vi "Homing.vi"(7 "Offset Home 2 RCM":dbl[](array[numeric])=[0.0, 0.0, 0.0, 0.0], 8 "error in":errorcluster, 9 "Stage PID Cluster":T2={"Stage Z PID"={"Kp"=0.0005, "Kd"=0.001, "Ki"=0.0}, "Stage Y PID"={"Kp"=0.0003, "Kd"=0.01, "Ki"=0.0}, "Stage X PID"={"Kp"=0.0003, "Kd"=0.01, "Ki"=0.0}}, 10 "L1 to L4 PID Cluster":T1={"L1 PID Gains"={"Kp"=0.005, "Kd"=0.5, "Ki"=0.0005}, "L2 PID Gains"={"Kp"=0.01, "Kd"=1.0, "Ki"=0.005}, "L3 PID Gains"={"Kp"=0.05, "Kd"=1.0, "Ki"=0.0005}, "L4 PID Gains"={"Kp"=0.1, "Kd"=0.1, "Ki"=0.0005}}, 11 "FPGA VI Reference In":refnum<k20>) -> (0 "error out":errorcluster, 1 "Last Stage Posit":dbl[](array[numeric]), 2 "Last L1 to L4 Posit":dbl[](array[numeric]), 3 "FPGA VI Reference Out":refnum<k20>)   [LabVIEW 2016]
uses:
  <vilib>/Platform/TimedLoop/XDataNode/timing_clust.ctl
  <vilib>/Platform/TimedLoop/XDataNode/nitl_modes.ctl
  <vilib>/Platform/TimedLoop/XDataNode/wakeup.ctl
  Library/KevinLibraryAll/labview2010/kevLib2010/Simple Filters/kDelay.vi
  Global Variables.vi
  <vilib>/Utility/error.llb/Error Cluster From Error Code.vi
  <vilib>/rvi/errors/niLvFpgaAdjustHostInterfaceError.vi
  <vilib>/platform/TimedLoop/XDataNode/XDataNode.xnode
  <vilib>/rvi/interface/nirviReadWriteControl/nirviReadWriteControl.xnode
  FPGA Bitfiles/PhantomControlPI_FPGATarget_QuadCtr2_E2412E44.lvbitx
  IRISS_FPGA_IO.vi
  <vilib>/Platform/TimedLoop/XDataNode/XDNodeRunTimeDep.lvlib
  Library/KevinLibraryAll/labview2010/kevLib2010.lvlib
  Library/KevinLibraryAll/labview2011/kevLib2011.lvlib
  Library/KevinLibraryAll/labview/KevLib01.lvlib
  Library/jmslib.lvlib
  NiFpgaLv.dll
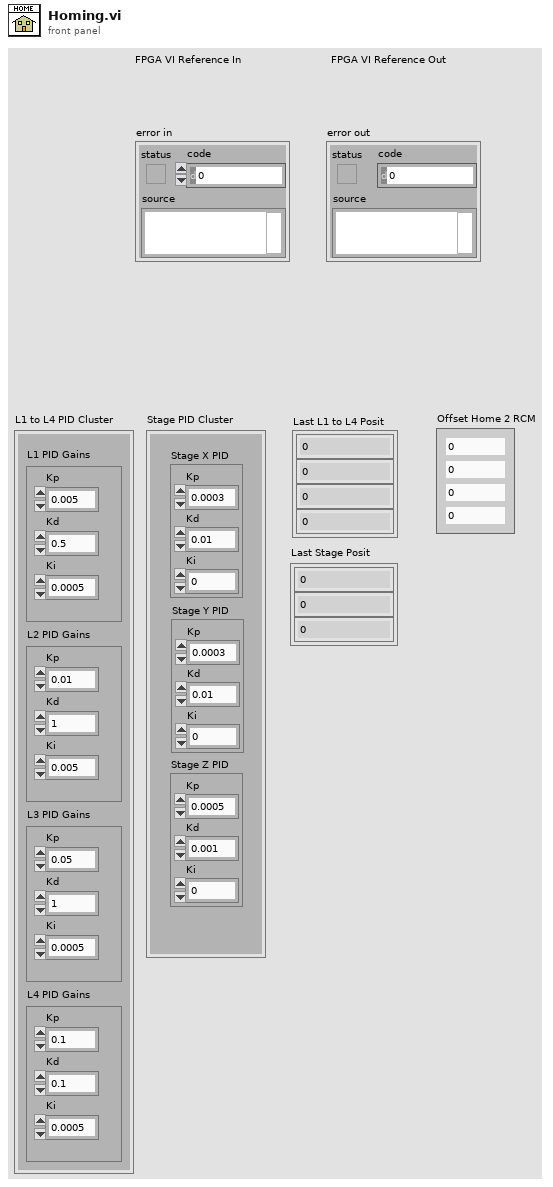
[diagram p1: front panel]
types:
  T1 = cluster{"L1 PID Gains":cluster{"Kp":dbl, "Kd":dbl, "Ki":dbl}, "L2 PID Gains":cluster{"Kp":dbl, "Kd":dbl, "Ki":dbl}, "L3 PID Gains":cluster{"Kp":dbl, "Kd":dbl, "Ki":dbl}, "L4 PID Gains":cluster{"Kp":dbl, "Kd":dbl, "Ki":dbl}}
  T2 = cluster{"Stage Z PID":cluster{"Kp":dbl, "Kd":dbl, "Ki":dbl}, "Stage Y PID":cluster{"Kp":dbl, "Kd":dbl, "Ki":dbl}, "Stage X PID":cluster{"Kp":dbl, "Kd":dbl, "Ki":dbl}}
  T3 = typedef "XDNodeRunTimeDep.lvlib/timing_clust.ctl" = cluster{"Expected End [f-1]":u64, "Actual End [f-1]":u64, "Finished Late? [f-1]":bool, "Expected End [i-1]":u64, "Actual End [i-1]":u64, "Finished Late? [i-1]":bool, "Expected Start [i]":u64, "Actual Start [i]":u64, "Expected Start [f]":u64, "Actual Start [f]":u64, "Source Name":string, "Structure Name":string, "Period":i64, "Deadline":i64, "Offset":i64, "Start":i64, "Priority":i32, "Timeout":i32, "Mode":T4, "Wakeup Reason":T5, "Error":errorcluster, "Source Type":string, "Secondary Source Type":string, "Global End Time":u64, "Global Start Time":u64, "Frame Duration":u64, "Iteration Duration":u64, "Assigned CPU":i32, "I/O Scan Engine Mode":u32}
  T4 = typedef "XDNodeRunTimeDep.lvlib/nitl_modes.ctl" = enum32{"No Change", "Process missed periods, maintain original phase", "Discard missed periods, maintain original phase", "Process missed periods, ignore original phase", "Discard missed periods, ignore original phase"}
  T5 = typedef "XDNodeRunTimeDep.lvlib/wakeup.ctl" = enum32{"Normal", "Aborted", "Asynchronous wakeup", "Timing source error", "Timed loop error", "Timeout"}
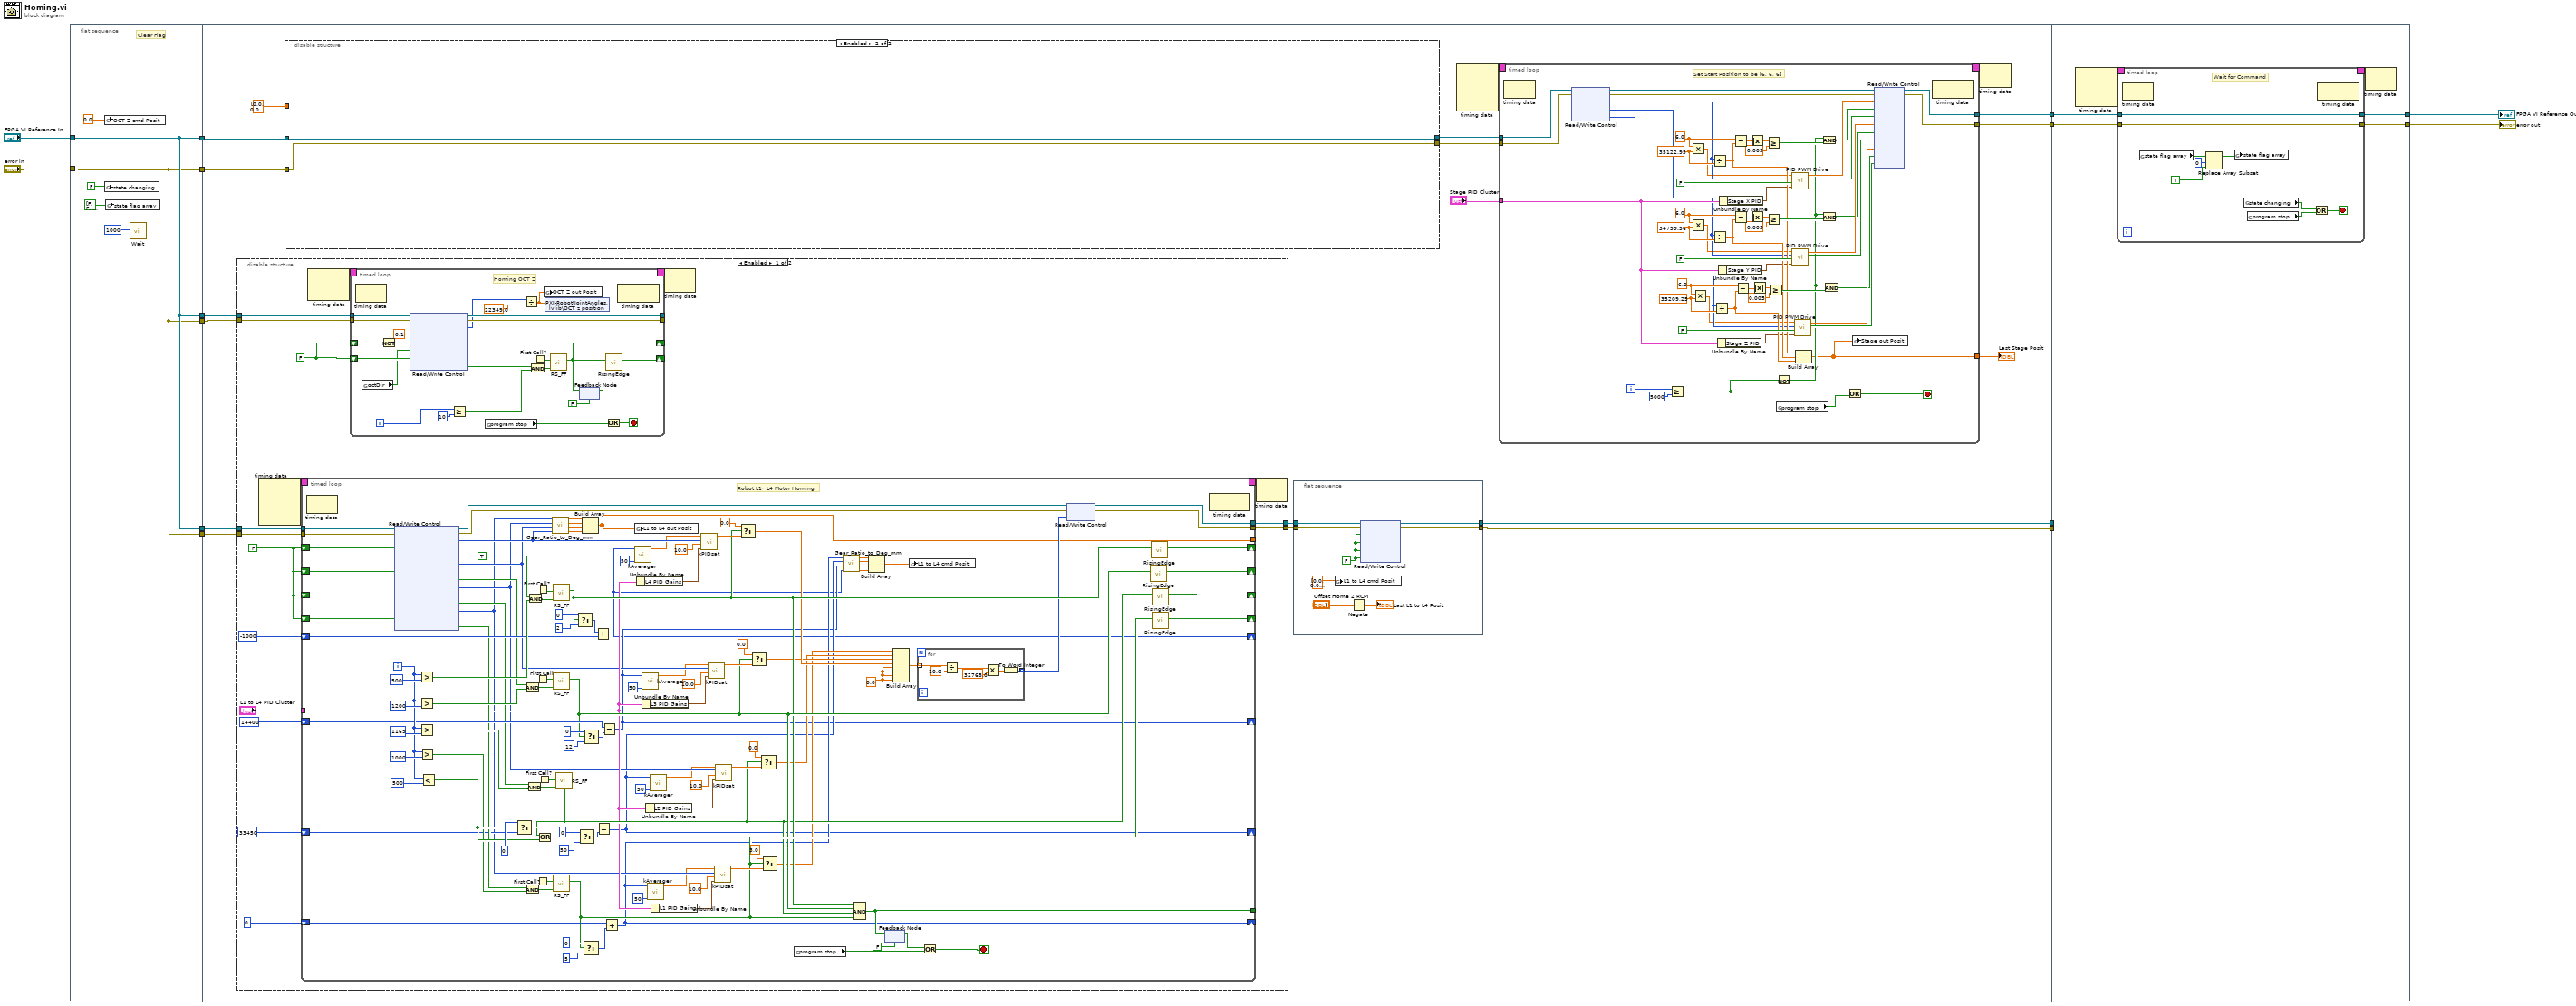
[diagram p0: block diagram]
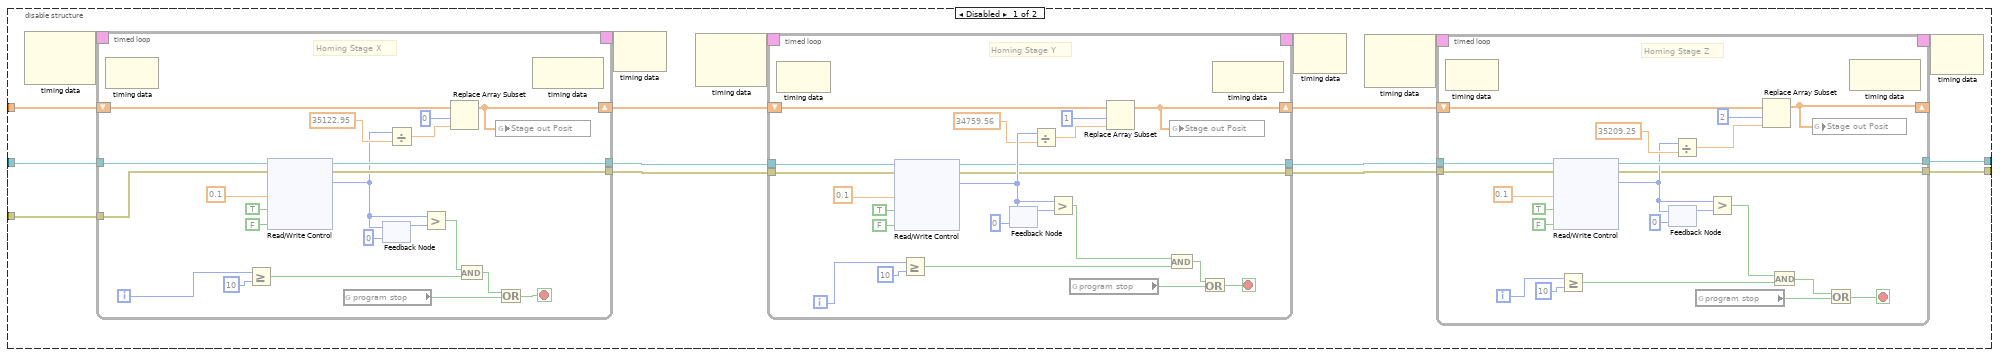
[diagram p3: hidden frame]
diagram:
  n1 = flat-sequence {
    tunnel: "FPGA VI Reference In" -> [w17]
    tunnel: "error in" -> [w16]
    tunnel: [w17] -> w14
    tunnel: [w17] -> w13
    tunnel: [w16] -> w12
    tunnel: [w16] -> w11
    tunnel: [w17] -> w6
    tunnel: [w16] -> w5
    tunnel: w14 -> [w37]
    tunnel: w13 -> [w36]
    tunnel: w12 -> [w35]
    tunnel: w11 -> [w34]
    tunnel: w6 -> [w33]
    tunnel: w5 -> [w32]
    tunnel: [w31] -> w4
    tunnel: [w30] -> w3
    tunnel: [w24] -> w2
    tunnel: [w23] -> w1
    tunnel: [w378] -> w8
    tunnel: [w377] -> w7
    tunnel: w4 -> [_]
    tunnel: w3 -> [_]
    tunnel: w2 -> [w376]
    tunnel: w1 -> [w375]
    frame #0 {
      # "Clear Flag"
      n2 = global write "Global Variables.vi" "OCT Z cmd Posit"(0.0) -> ()
      n3 = global write "Global Variables.vi" "state changing"(FALSE ("state changing")) -> ()
      n4 = global write "Global Variables.vi" "state flag array"(bool[] [FALSE, FALSE, FALSE, FALSE, FALSE, FALSE, FALSE, FALSE, FALSE] ("state flag array")) -> ()
      n5 = call "Wait"("Count(mSec)"=u32 1000 ("milliseconds to wait")) -> ()  [unwired: 1 out]
    }
    frame #1 {
      n6 = disable-structure shown="Enabled" {
        disable-tunnel: w36 -> [w52 _]
        disable-tunnel: w34 -> [w51 _]
        disable-tunnel: w33 -> [w50 _]
        disable-tunnel: w32 -> [w49 _]
        disable-tunnel: [w47 _] -> w22
        disable-tunnel: [w46 _] -> w21
        frame Enabled {
          w45 = FALSE ("Rising Edge")
          w48 = FALSE ("Rising Edge")
          n7 = node-c288() -> (w54:T3)  [unwired: 4 in]
          n8 = timed-loop {
            timing: w54 -> [_]
            timing-out: [_] -> w53
            tunnel: w52 -> [w171]
            tunnel: w51 -> [w170]
            shift-right: [w105] -> _
            shift-left: w45 -> [w169]
            shift-right: [w104] -> _
            shift-left: w45 -> [w168]
            shift-right: [w103] -> _
            shift-left: w45 -> [w167]
            shift-right: [w102] -> _
            shift-left: w45 -> [w166]
            shift-right: [w60] -> _
            shift-left: -1000 -> [w149]
            shift-right: [w61] -> _
            shift-left: 14400 -> [w141]
            shift-right: [w62] -> _
            shift-left: 33450 -> [w112]
            shift-right: [w63] -> _
            shift-left: 0 -> [w111]
            tunnel: [w106] -> _
            tunnel: [w86] -> w47
            tunnel: [w85] -> w46
            tunnel: "L1 to L4 PID Cluster" -> [w81]
            tunnel: [w59] -> _
            i -> [w151]
            stop <- w107 stop-if-true
            w97 = 0.0 ("element")
            # "Robot L1~L4 Motor Homing"
            n9 = node-c288() -> ()  [unwired: 1 in, 1 out]
            n10 = xnode "Read/Write Control"("FPGA VI Reference In"=w171, "error in"=w170, "Reset C1-4"=w169, "Reset C1-1"=w168, "Reset 3"=w167, "Reset 1"=w166) -> ("FPGA VI Reference Out"=w94:refnum<k20>, "error out"=w93:errorcluster, "32 bit Position C1-4"=w79:i32, "32 bit Position C1-1"=w78:i32, "Home L3"=w132:bool, "32 bit Position 3"=w77:i32, "Home L2"=w130:bool, "32 bit Position 1"=w76:i32, "Home L1"=w117:bool)  [unwired: 1 out]
            n11 = Greater?(x=w151, y=500) -> (0:w150:bool)
            n12 = Greater?(x=w151, y=1200) -> (0:w133:bool)
            n13 = Greater?(x=w151, y=1169) -> (0:w131:bool)
            n14 = Greater?(x=w151, y=1000) -> (0:w116:bool)
            n15 = Less?(x=w151, y=500) -> (x < y?=w123:bool)
            n16 = Select(t=0, s=w123, f=w112) -> (s? t:f=w128:i32)
            n17 = And(x=w132, y=w133) -> (x .and. y?=w142:bool)
            n18 = And(x=w117, y=w116) -> (x .and. y?=w118:bool)
            n19 = And(x=w130, y=w131) -> (x .and. y?=w135:bool)
            n20 = And(x=TRUE, y=w150) -> (x .and. y?=w162:bool)
            n21 = First Call?() -> (First Call?: T/F=w143:bool)
            n22 = First Call?() -> (First Call?: T/F=w119:bool)
            n23 = First Call?() -> (First Call?: T/F=w161:bool)
            n24 = First Call?() -> (First Call?: T/F=w134:bool)
            n25 = call "Gear_Ratio_to_Deg_mm.vi"("j4"=w79, "j3"=w78, "j2"=w77, "j1"=w76) -> ("theta 4"=w72:dbl, "theta 3"=w73:dbl, "theta 2"=w74:dbl, "theta 1"=w75:dbl)
            n26 = call "RS_FF.vi"("Set"=w162, "Reset"=w161) -> ("Result"=w99:bool)  [unwired: 9 in]
            n27 = call "RS_FF.vi"("Set"=w142, "Reset"=w143) -> ("Result"=w100:bool)  [unwired: 9 in]
            n28 = call "RS_FF.vi"("Set"=w118, "Reset"=w119) -> ("Result"=w101:bool)  [unwired: 9 in]
            n29 = call "RS_FF.vi"("Set"=w135, "Reset"=w134) -> ("Result"=w98:bool)  [unwired: 9 in]
            n30 = Or(x=w98, y=w123) -> (x .or. y?=w127:bool)
            n31 = Select(t=0, s=w99, f=2) -> (s? t:f=w163:i32)
            n32 = Select(t=0, s=w127, f=50) -> (s? t:f=w124:i32)
            n33 = Build Array(w75, w74, w73, w72) -> (w59:dbl[])
            n34 = Select(t=0, s=w101, f=5) -> (s? t:f=w122:i32)
            n35 = Select(t=0, s=w100, f=12) -> (s? t:f=w144:i32)
            n36 = Add(x=w163, y=w149) -> (x+y=w60:i32)
            n37 = Subtract(x=w128, y=w124) -> (x-y=w62:i32)
            n38 = Subtract(x=w141, y=w144) -> (x-y=w61:i32)
            n39 = Add(x=w111, y=w122) -> (x+y=w63:i32)
            n40 = call "kAverager.vi"("num avg"=50, "input"=w60) -> ("output"=w64:dbl)  [unwired: 9 in]
            n41 = global write "Global Variables.vi" "L1 to L4 out Posit"(w59) -> ()
            n42 = Unbundle By Name(w81) -> ("L4 PID Gains"=w84:cluster{"Kp":dbl, "Kd":dbl, "Ki":dbl})
            n43 = Unbundle By Name(w81) -> ("L3 PID Gains"=w83:cluster{"Kp":dbl, "Kd":dbl, "Ki":dbl})
            n44 = call "kAverager.vi"("num avg"=50, "input"=w61) -> ("output"=w65:dbl)  [unwired: 9 in]
            n45 = Unbundle By Name(w81) -> ("L2 PID Gains"=w82:cluster{"Kp":dbl, "Kd":dbl, "Ki":dbl})
            n46 = call "kAverager.vi"("num avg"=50, "input"=w63) -> ("output"=w67:dbl)  [unwired: 9 in]
            n47 = call "kAverager.vi"("num avg"=50, "input"=w62) -> ("output"=w66:dbl)  [unwired: 9 in]
            n48 = Unbundle By Name(w81) -> ("L1 PID Gains"=w80:cluster{"Kp":dbl, "Kd":dbl, "Ki":dbl})
            n49 = call "kPIDsat.vi"("PID Gains"=w84, "Sat Limit"=10.0, "Position"=w79, "Reference"=w64) -> ("Control"=w158:dbl)  [unwired: 7 in]
            n50 = call "kPIDsat.vi"("PID Gains"=w83, "Sat Limit"=10.0, "Position"=w78, "Reference"=w65) -> ("Control"=w139:dbl)  [unwired: 7 in]
            n51 = call "kPIDsat.vi"("PID Gains"=w80, "Sat Limit"=10.0, "Position"=w76, "Reference"=w67) -> ("Control"=w113:dbl)  [unwired: 7 in]
            n52 = call "kPIDsat.vi"("PID Gains"=w82, "Sat Limit"=10.0, "Position"=w77, "Reference"=w66) -> ("Control"=w138:dbl)  [unwired: 7 in]
            n53 = Select(t=0.0, s=w99, f=w158) -> (s? t:f=w92:dbl)
            n54 = Select(t=0.0 ("element"), s=w100, f=w139) -> (s? t:f=w91:dbl)
            n55 = Select(t=0.0 ("element"), s=w98, f=w138) -> (s? t:f=w90:dbl)
            n56 = Select(t=3.0 ("element"), s=w101, f=w113) -> (s? t:f=w89:dbl)
            n57 = global read "Global Variables.vi" "program stop"() -> (w108:bool)
            n58 = call "Gear_Ratio_to_Deg_mm.vi"("j4"=w60, "j3"=w61, "j2"=w62, "j1"=w63) -> ("theta 4"=w68:dbl, "theta 3"=w69:dbl, "theta 2"=w70:dbl, "theta 1"=w71:dbl)
            n59 = Compound Arithmetic op=AND(w99, w100, w98, w101) -> (w106:bool)
            n60 = Build Array(w71, w70, w69, w68) -> (w58:dbl[])
            n61 = feedback #1(FALSE) -> (w109:bool)
            n62 = feedback-in #1(w106) -> ()
            n63 = Build Array(w89, w90, w91, w92, w97, w97, w97, w97) -> (w96:dbl[])
            n64 = global write "Global Variables.vi" "L1 to L4 cmd Posit"(w58) -> ()
            n65 = for {
              tunnel: [w175] -> w95 mode=indexing
              tunnel: w96 -> [w174] mode=indexing
              n66 = Divide(x=w174, y=10.0) -> (x/y=w177:dbl)
              n67 = Multiply(x=w177, y=32768.0) -> (x*y=w176:dbl)
              n68 = To Word Integer(number=w176) -> (16bit integer=w175:i16)
            }
            n69 = Or(x=w109, y=w108) -> (x .or. y?=w107:bool)
            n70 = xnode "Read/Write Control"("FPGA VI Reference In"=w94, "error in"=w93, "AO"=w95) -> ("FPGA VI Reference Out"=w86:refnum<k20>, "error out"=w85:errorcluster)
            n71 = call "RisingEdge.vi"("Signal In"=w100) -> ("Rising Edge"=w104:bool)  [unwired: 10 in]
            n72 = call "RisingEdge.vi"("Signal In"=w99) -> ("Rising Edge"=w105:bool)  [unwired: 10 in]
            n73 = call "RisingEdge.vi"("Signal In"=w98) -> ("Rising Edge"=w103:bool)  [unwired: 10 in]
            n74 = call "RisingEdge.vi"("Signal In"=w101) -> ("Rising Edge"=w102:bool)  [unwired: 10 in]
            n75 = node-c288() -> ()  [unwired: 1 in, 1 out]
          }
          n76 = node-c288() -> (w56:T3)  [unwired: 2 in]
          n77 = timed-loop {
            timing: w56 -> [_]
            timing-out: [_] -> w55
            tunnel: w50 -> [w202]
            tunnel: w49 -> [w201]
            tunnel: [w200] -> _
            tunnel: [w199] -> _
            shift-right: [w194] -> _
            shift-left: w48 -> [w196]
            shift-right: [w190] -> _
            shift-left: w48 -> [w188]
            i -> [w203]
            stop <- w197 stop-if-true
            # "Homing OCT Z"
            n78 = node-c288() -> ()  [unwired: 1 in, 1 out]
            n79 = global read "Global Variables.vi" "octDir"() -> (w182:bool)
            n80 = Not(x=w188) -> (.not. x?=w187:bool)
            n81 = xnode "Read/Write Control"("FPGA VI Reference In"=w202, "error in"=w201, "OCT Mot DC"=0.1 ("y"), "INHB OCT Mot"=w187, "DIR OCT Mot"=w182, "Reset 14"=w196) -> ("FPGA VI Reference Out"=w200:refnum<k20>, "error out"=w199:errorcluster, "32 bit Position 14"=w185:i32, "Home OCT z"=w195:bool)
            n82 = Greater Or Equal?(x=w203, y=10) -> (x >= y?=w205:bool)
            n83 = global read "Global Variables.vi" "program stop"() -> (w198:bool)
            n84 = Divide(x=w185, y=22349.0) -> (x/y=w183:dbl)
            n85 = And(x=w195, y=w205) -> (x .and. y?=w192:bool)
            n86 = First Call?() -> (First Call?: T/F=w193:bool)
            n87 = global write "Global Variables.vi" "OCT Z out Posit"(w183) -> ()
            n88 = shared-variable "PXI-Robot\\JointAngles.lvlib\\OCT z position"(w183) -> ()  [unwired: 1 in, 1 out]
            n89 = call "RS_FF.vi"("Set"=w192, "Reset"=w193) -> ("Result"=w190:bool)  [unwired: 9 in]
            n90 = feedback #2(FALSE) -> (w189:bool)
            n91 = feedback-in #2(w190) -> ()
            n92 = call "RisingEdge.vi"("Signal In"=w190) -> ("Rising Edge"=w194:bool)  [unwired: 10 in]
            n93 = Or(x=w189, y=w198) -> (x .or. y?=w197:bool)
            n94 = node-c288() -> ()  [unwired: 1 in, 1 out]
          }
          n95 = node-c288(w55) -> ()  [unwired: 1 out]
          n96 = node-c288(w53) -> ()  [unwired: 1 out]
        }
        frame Disabled {
        }
      }
      n97 = disable-structure shown="Enabled" {
        disable-tunnel: [w220 w306] -> w39
        disable-tunnel: [w219 w305] -> w38
        disable-tunnel: w37 -> [w218 w306]
        disable-tunnel: w35 -> [w217 w305]
        disable-tunnel: dbl[] [0.0, 0.0, 0.0] ("Stage Posit Array") -> [w210 _]
        frame Disabled {
          n98 = node-c288() -> (w222:T3)  [unwired: 2 in]
          n99 = timed-loop {
            timing: w222 -> [_]
            timing-out: [_] -> w221
            tunnel: w218 -> [w238]
            tunnel: w217 -> [w237]
            tunnel: [w236] -> w213
            tunnel: [w235] -> w212
            shift-right: [w227] -> w211
            shift-left: w210 -> [w229]
            i -> [w239]
            stop <- w232 stop-if-true
            # "Homing Stage X"
            n100 = node-c288() -> ()  [unwired: 1 in, 1 out]
            n101 = Greater Or Equal?(x=w239, y=10) -> (x >= y?=w248:bool)
            n102 = xnode "Read/Write Control"("FPGA VI Reference In"=w238, "error in"=w237, "X DC"=0.1 ("y"), "INHB X"=TRUE ("INHB Y"), "DIR X"=FALSE ("INHB Y")) -> ("FPGA VI Reference Out"=w236:refnum<k20>, "error out"=w235:errorcluster, "Position X"=w228:i32)
            n103 = global read "Global Variables.vi" "program stop"() -> (w234:bool)
            n104 = feedback #3(0 ("Position Y")) -> (w245:i32)
            n105 = feedback-in #3(w228) -> ()
            n106 = Divide(x=w228, y=35122.95) -> (x/y=w230:dbl)
            n107 = Greater?(x=w228, y=w245) -> (0:w246:bool)
            n108 = Replace Array Subset(array=w229, new element=w230, index=0) -> (w227:dbl[])
            n109 = And(x=w246, y=w248) -> (x .and. y?=w233:bool)
            n110 = global write "Global Variables.vi" "Stage out Posit"(w227) -> ()
            n111 = Or(x=w233, y=w234) -> (x .or. y?=w232:bool)
            n112 = node-c288() -> ()  [unwired: 1 in, 1 out]
          }
          n113 = node-c288(w221) -> ()  [unwired: 1 out]
          n114 = node-c288() -> (w224:T3)  [unwired: 2 in]
          n115 = timed-loop {
            timing: w224 -> [_]
            timing-out: [_] -> w223
            tunnel: w213 -> [w263]
            tunnel: w212 -> [w264]
            tunnel: [w261] -> w216
            tunnel: [w260] -> w215
            shift-right: [w253] -> w214
            shift-left: w211 -> [w254]
            i -> [w262]
            stop <- w259 stop-if-true
            # "Homing Stage Y"
            n116 = node-c288() -> ()  [unwired: 1 in, 1 out]
            n117 = xnode "Read/Write Control"("FPGA VI Reference In"=w263, "error in"=w264, "Y DC"=0.1 ("y"), "INHB Y"=TRUE, "DIR Y"=FALSE ("INHB Y")) -> ("FPGA VI Reference Out"=w261:refnum<k20>, "error out"=w260:errorcluster, "Position Y"=w271:i32)
            n118 = Greater Or Equal?(x=w262, y=10) -> (x >= y?=w274:bool)
            n119 = feedback #4(0 ("Position Y")) -> (w270:i32)
            n120 = feedback-in #4(w271) -> ()
            n121 = Divide(x=w271, y=34759.56) -> (x/y=w255:dbl)
            n122 = Greater?(x=w271, y=w270) -> (0:w272:bool)
            n123 = global read "Global Variables.vi" "program stop"() -> (w257:bool)
            n124 = Replace Array Subset(array=w254, new element=w255, index=1) -> (w253:dbl[])
            n125 = And(x=w272, y=w274) -> (x .and. y?=w258:bool)
            n126 = global write "Global Variables.vi" "Stage out Posit"(w253) -> ()
            n127 = Or(x=w258, y=w257) -> (x .or. y?=w259:bool)
            n128 = node-c288() -> ()  [unwired: 1 in, 1 out]
          }
          n129 = node-c288(w223) -> ()  [unwired: 1 out]
          n130 = node-c288() -> (w226:T3)  [unwired: 2 in]
          n131 = timed-loop {
            timing: w226 -> [_]
            timing-out: [_] -> w225
            tunnel: w216 -> [w300]
            tunnel: [w299] -> w220
            tunnel: w215 -> [w287]
            tunnel: [w286] -> w219
            shift-right: [w279] -> _
            shift-left: w214 -> [w280]
            i -> [w290]
            stop <- w284 stop-if-true
            # "Homing Stage Z"
            n132 = node-c288() -> ()  [unwired: 1 in, 1 out]
            n133 = xnode "Read/Write Control"("FPGA VI Reference In"=w300, "error in"=w287, "Z DC"=0.1 ("y"), "INHB Z"=TRUE ("INHB Y"), "DIR Z"=FALSE ("INHB Y")) -> ("FPGA VI Reference Out"=w299:refnum<k20>, "error out"=w286:errorcluster, "Position Z"=w292:i32)
            n134 = Greater Or Equal?(x=w290, y=10) -> (x >= y?=w288:bool)
            n135 = feedback-in #5(w292) -> ()
            n136 = feedback #5(0 ("Position Y")) -> (w293:i32)
            n137 = Divide(x=w292, y=35209.25) -> (x/y=w281:dbl)
            n138 = global read "Global Variables.vi" "program stop"() -> (w285:bool)
            n139 = Greater?(x=w292, y=w293) -> (0:w291:bool)
            n140 = Replace Array Subset(array=w280, new element=w281, index=2) -> (w279:dbl[])
            n141 = And(x=w291, y=w288) -> (x .and. y?=w283:bool)
            n142 = global write "Global Variables.vi" "Stage out Posit"(w279) -> ()
            n143 = Or(x=w283, y=w285) -> (x .or. y?=w284:bool)
            n144 = node-c288() -> ()  [unwired: 1 in, 1 out]
          }
          n145 = node-c288(w225) -> ()  [unwired: 1 out]
        }
        frame Enabled {
        }
      }
      n146 = flat-sequence {
        tunnel: w22 -> [w313]
        tunnel: w21 -> [w312]
        tunnel: [w308] -> w31
        tunnel: [w307] -> w30
        frame #0 {
          w314 = FALSE ("Reset 1")
          n147 = global write "Global Variables.vi" "L1 to L4 cmd Posit"(dbl[] [0.0, 0.0, 0.0, 0.0] ("L1 to L4 cmd Posit")) -> ()
          n148 = Negate(x="Offset Home 2 RCM") -> (-x=→"Last L1 to L4 Posit":dbl[])
          n149 = xnode "Read/Write Control"("FPGA VI Reference In"=w313, "error in"=w312, "Reset C1-4"=w314, "Reset C1-1"=w314, "Reset 3"=w314, "Reset 1"=w314) -> ("FPGA VI Reference Out"=w308:refnum<k20>, "error out"=w307:errorcluster)
        }
      }
      n150 = node-c288() -> (w29:T3)  [unwired: 4 in]
      n151 = timed-loop {
        timing: w29 -> [_]
        timing-out: [_] -> w28
        tunnel: w39 -> [w335]
        tunnel: w38 -> [w336]
        tunnel: "Stage PID Cluster" -> [w344]
        tunnel: [w317] -> w26
        tunnel: [w316] -> w24
        tunnel: [w315] -> w23
        i -> [w370]
        stop <- w334 stop-if-true
        w347 = 6.0 ("y")
        w350 = 35209.25 ("y")
        w361 = 6.0 ("y")
        w358 = 34759.56 ("y")
        w362 = 6.0 ("y")
        w365 = 35122.95 ("y")
        # "Set Start Position to be [6, 6, 6]"
        n152 = node-c288() -> ()  [unwired: 1 in, 1 out]
        n153 = xnode "Read/Write Control"("FPGA VI Reference In"=w335, "error in"=w336) -> ("FPGA VI Reference Out"=w338:refnum<k20>, "error out"=w337:errorcluster, "Position X"=w333:i32, "Position Y"=w332:i32, "Position Z"=w331:i32)
        n154 = Greater Or Equal?(x=w370, y=5000) -> (x >= y?=w323:bool)
        n155 = Multiply(x=w362, y=w365) -> (x*y=w330:dbl)
        n156 = Multiply(x=w361, y=w358) -> (x*y=w329:dbl)
        n157 = Multiply(x=w347, y=w350) -> (x*y=w328:dbl)
        n158 = Divide(x=w333, y=w365) -> (x/y=w343:dbl)
        n159 = Divide(x=w332, y=w358) -> (x/y=w342:dbl)
        n160 = Divide(x=w331, y=w350) -> (x/y=w341:dbl)
        n161 = Unbundle By Name(w344) -> ("Stage Z PID"=w339:cluster{"Kp":dbl, "Kd":dbl, "Ki":dbl})
        n162 = Unbundle By Name(w344) -> ("Stage Y PID"=w340:cluster{"Kp":dbl, "Kd":dbl, "Ki":dbl})
        n163 = Unbundle By Name(w344) -> ("Stage X PID"=w324:cluster{"Kp":dbl, "Kd":dbl, "Ki":dbl})
        n164 = Subtract(x=w362, y=w343) -> (x-y=w366:dbl)
        n165 = Subtract(x=w361, y=w342) -> (x-y=w357:dbl)
        n166 = Subtract(x=w347, y=w341) -> (x-y=w351:dbl)
        n167 = Absolute Value(x=w366) -> (abs(x)=w367:dbl)
        n168 = Absolute Value(x=w357) -> (abs(x)=w356:dbl)
        n169 = Absolute Value(x=w351) -> (abs(x)=w352:dbl)
        n170 = Greater Or Equal?(x=w367, y=0.005) -> (x >= y?=w363:bool)
        n171 = Greater Or Equal?(x=w356, y=0.005) -> (x >= y?=w360:bool)
        n172 = Greater Or Equal?(x=w352, y=0.005) -> (x >= y?=w348:bool)
        n173 = Not(x=w323) -> (.not. x?=w322:bool)
        n174 = global read "Global Variables.vi" "program stop"() -> (w345:bool)
        n175 = call "PID PWM Drive.vi"("PID Gains"=w324, "Reverse Motor?"=FALSE, "Encoder Position"=w333, "Reference"=w330) -> ("Direction"=w320:bool, "Duty Cycle"=w327:dbl)  [unwired: 5 in, 1 out]
        n176 = call "PID PWM Drive.vi"("PID Gains"=w340, "Reverse Motor?"=FALSE, "Encoder Position"=w332, "Reference"=w329) -> ("Direction"=w354:bool, "Duty Cycle"=w326:dbl)  [unwired: 5 in, 1 out]
        n177 = call "PID PWM Drive.vi"("PID Gains"=w339, "Reverse Motor?"=FALSE, "Encoder Position"=w331, "Reference"=w328) -> ("Direction"=w346:bool, "Duty Cycle"=w325:dbl)  [unwired: 5 in, 1 out]
        n178 = Build Array(w343, w342, w341) -> (w317:dbl[])
        n179 = And(x=w322, y=w363) -> (x .and. y?=w321:bool)
        n180 = And(x=w322, y=w360) -> (x .and. y?=w319:bool)
        n181 = And(x=w322, y=w348) -> (x .and. y?=w318:bool)
        n182 = Or(x=w323, y=w345) -> (x .or. y?=w334:bool)
        n183 = global write "Global Variables.vi" "Stage out Posit"(w317) -> ()
        n184 = xnode "Read/Write Control"("FPGA VI Reference In"=w338, "error in"=w337, "X DC"=w327, "INHB X"=w321, "DIR X"=w320, "Y DC"=w326, "INHB Y"=w319, "DIR Y"=w354, "Z DC"=w325, "INHB Z"=w318, "DIR Z"=w346) -> ("FPGA VI Reference Out"=w316:refnum<k20>, "error out"=w315:errorcluster)
        n185 = node-c288() -> ()  [unwired: 1 in, 1 out]
      }
      "Last Stage Posit" <- w26
      n186 = node-c288(w28) -> ()  [unwired: 1 out]
    }
    frame #2 {
      n187 = node-c288() -> (w380:T3)  [unwired: 3 in]
      n188 = timed-loop {
        timing: w380 -> [_]
        timing-out: [_] -> w379
        tunnel: w376 -> [w383]
        tunnel: [w383] -> w378
        tunnel: [w382] -> w377
        tunnel: w375 -> [w382]
        stop <- w381 stop-if-true
        # "Wait for Command"
        n189 = node-c288() -> ()  [unwired: 1 in, 1 out]
        n190 = global read "Global Variables.vi" "state flag array"() -> (w387:bool[])
        n191 = Replace Array Subset(array=w387, new element=TRUE ("new element/subarray"), index=0) -> (w386:bool[])
        n192 = global write "Global Variables.vi" "state flag array"(w386) -> ()
        n193 = global read "Global Variables.vi" "state changing"() -> (w389:bool)
        n194 = global read "Global Variables.vi" "program stop"() -> (w388:bool)
        n195 = Or(x=w389, y=w388) -> (x .or. y?=w381:bool)
        n196 = node-c288() -> ()  [unwired: 1 in, 1 out]
      }
      n197 = node-c288(w379) -> ()  [unwired: 1 out]
    }
  }
  "FPGA VI Reference Out" <- w8
  "error out" <- w7
